vi "Add Sub Object.vi"(8 "error in":errorcluster, 10 "Sub Object":refnum<class "Sub Object.lvclass">, 11 "Object Dictionary in":refnum<class "Object Dictionary.lvclass">) -> (0 "error out":errorcluster, 2 "Success":bool, 3 "Object Dictionary out":refnum<class "Object Dictionary.lvclass">)   [LabVIEW 2019, in "Electronic Datasheet.lvlib" / "Object Dictionary.lvclass"]
uses:
  Object Dictionary.lvclass
  Object Dictionary.lvclass/Object Dictionary.ctl
  Sub Object/Sub Object.lvclass
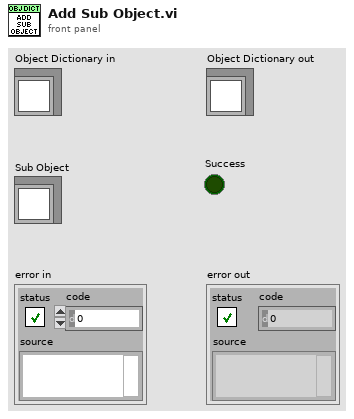
[diagram p1: front panel]
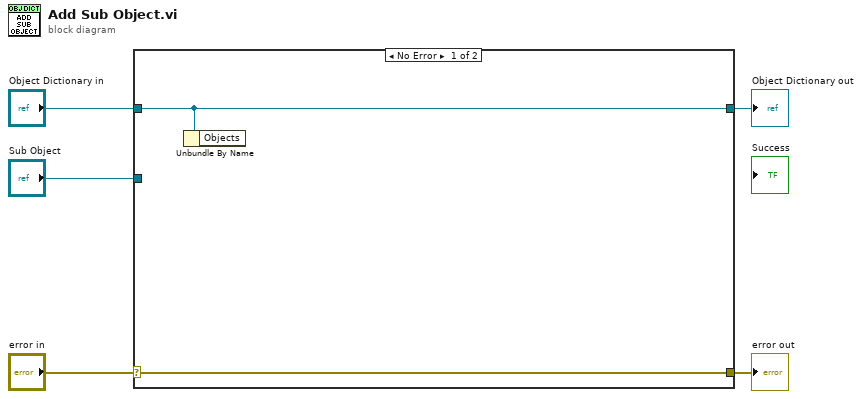
[diagram p0: block diagram]
diagram:
  n1 = case shown="No Error" "error in" {
    selector: "error in" -> [w7 w9]
    tunnel: [w7 w9] -> w4
    tunnel: [w6 w8] -> w2
    tunnel: "Object Dictionary in" -> [w6 w8]
    tunnel: "Sub Object" -> [_ _]
    frame No Error {
      n2 = Unbundle By Name(w6) -> ()  [unwired: 1 out]
    }
    frame Error {
    }
  }
  "error out" <- w4
  "Object Dictionary out" <- w2
